vi "WireNum2SpatialPos.vi"(11 "Waveforms":sgl[][](graph)) -> (3 "Peak Values":cluster{"Z Element Position":sgl[], sgl[]}[](graph))   [LabVIEW 2022 SP3]
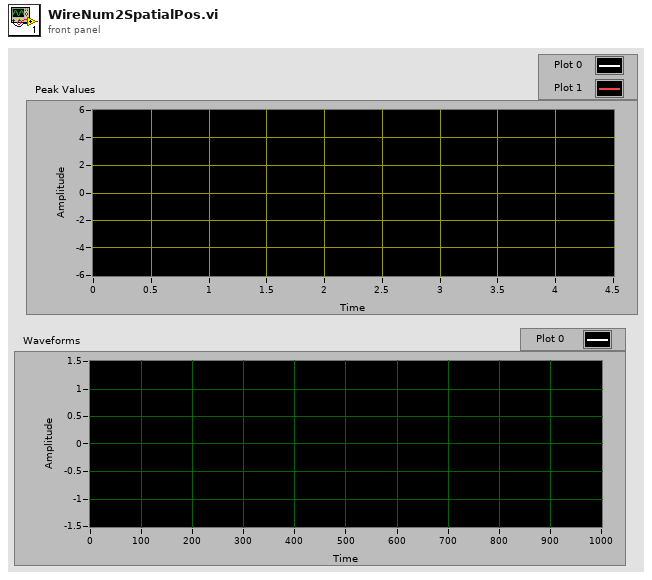
[diagram p1: front panel]
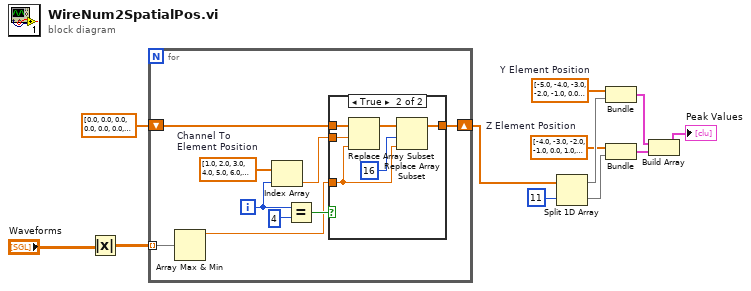
[diagram p0: block diagram]
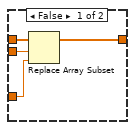
[diagram p2: hidden frame]
diagram:
  w3 = sgl[] [-4.0, -3.0, -2.0, -1.0, 0.0, 1.0, 2.0, 3.0, 4.0, 5.0]  # Z Element Position
  w4 = sgl[] [-5.0, -4.0, -3.0, -2.0, -1.0, 0.0, 1.0, 2.0, 3.0, 4.0, 5.0]  # Y Element Position
  n1 = Absolute Value(x="Waveforms") -> (abs(x)=w6:sgl[][])
  n2 = for {
    tunnel: w6 -> [w14] mode=indexing
    shift-right: [w18] -> w12
    shift-left: sgl[] [0.0, 0.0, 0.0, 0.0, 0.0, 0.0, 0.0, 0.0, 0.0, 0.0, 0.0, 0.0, 0.0, 0.0, 0.0, 0.0, 0.0, 0.0, 0.0, 0.0, 0.0, 0.0] ("Channel To \nElement Position") -> [w19]
    i -> [w15]
    w17 = sgl[] [1.0, 2.0, 3.0, 4.0, 5.0, 6.0, 7.0, 8.0, 9.0, 12.0, 13.0, 14.0, 16.0, 17.0, 18.0, 19.0, 0.0, 10.0, 11.0, 20.0]  # Channel To  Element Position
    n3 = Array Max & Min(array=w14) -> (max value=w13:sgl)  [unwired: 3 out]
    n4 = Index Array(array=w17, index=w15) -> (element=w16:sgl)
    n5 = Equal?(x=w15, y=4) -> (x = y?=w20:bool)
    n6 = case shown="True" w20 {
      tunnel: w19 -> [w24 w29]
      tunnel: w13 -> [w23 w28]
      tunnel: [w25 w27] -> w18
      tunnel: w16 -> [w22 w26]
      frame False {
        n7 = Replace Array Subset(array=w24, new element=w23, index=w22) -> (w25:sgl[])
      }
      frame True {
        n8 = Replace Array Subset(array=w29, new element=w28, index=w26) -> (w30:sgl[])
        n9 = Replace Array Subset(array=w30, new element=w28, index=16) -> (w27:sgl[])
      }
    }
  }
  n10 = Split 1D Array(array=w12, index=11) -> (first subarray=w5:sgl[], second subarray=w2:sgl[])
  n11 = Bundle("Y Element Position"=w4, w5) -> (w9:cluster{"Y Element Position":sgl[], sgl[]})  [unwired: 1 in]
  n12 = Bundle("Z Element Position"=w3, w2) -> (w8:cluster{"Z Element Position":sgl[], sgl[]})  [unwired: 1 in]
  n13 = Build Array(w9, w8) -> (→"Peak Values":cluster{"Z Element Position":sgl[], sgl[]}[])
